vi "Write TDMS File.vi"(8 "error in (no error)":errorcluster, 10 "Data":dbl[](array[numeric]), 11 "Path":path) -> (0 "error out":errorcluster)   [LabVIEW 2022 SP3]
uses:
  <vilib>/Utility/TDMS File Viewer/NI_TDMS File Viewer.lvlib
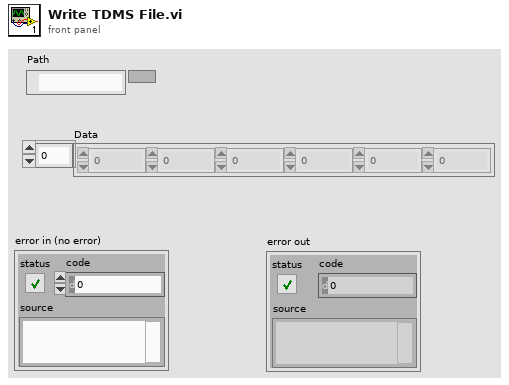
[diagram p1: front panel]
types:
  T1 = enum16{"open", "open or create", "create or replace", "create", "open (read-only)"}
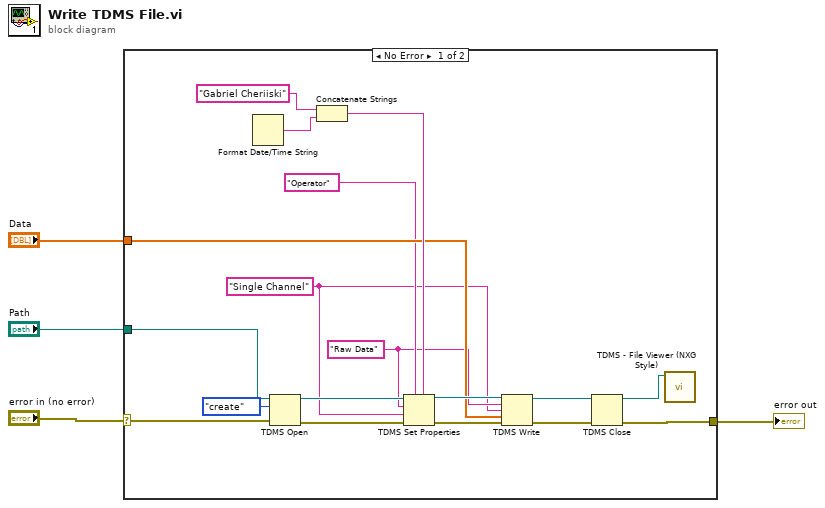
[diagram p0: block diagram]
diagram:
  n1 = case shown="No Error" "error in (no error)" {
    selector: "error in (no error)" -> [w20 w23]
    tunnel: [w16 w23] -> w3
    tunnel: "Path" -> [w15 _]
    tunnel: "Data" -> [w9 _]
    frame No Error {
      w6 = "Single Channel" ("channel name")
      w7 = "Raw Data" ("group name")
      n2 = Format Date/Time String() -> (date/time string=w21:string)  [unwired: 3 in]
      n3 = TDMS Open(8:w20, 10:T1."create" ("operation (0:open)"), 11:w15) -> (0:w19:errorcluster, 3:w14:refnum<k34>)  [unwired: 4 in]
      n4 = Concatenate Strings("Gabriel Cheriiski", w21) -> (w10:string)
      n5 = TDMS Set Properties(5:w10, 7:"Operator" ("property names"), 8:w19, 9:w6, 10:w7, 11:w14) -> (0:w18:errorcluster, 3:w13:refnum<k34>)  [unwired: 2 out]
      n6 = TDMS Write(0:w13, 5:w7, 7:w6, 9:w9, 11:w18) -> (4:w12:refnum<k34>, 15:w17:errorcluster)  [unwired: 1 in, 2 out]
      n7 = TDMS Close(8:w17, 11:w12) -> (0:w16:errorcluster, 3:w5:path)
      n8 = call <vilib>:"TDMS - File Viewer (NXG Style).vi"("file in"=w5) -> ()  [unwired: 9 in, 2 out]
    }
    frame Error {
    }
  }
  "error out" <- w3
